vi "Calculate Load Positons from Tube Positions.vi"(7 "PPR":i32=1024, 10 "Tube Counts":i32[](array[numeric])=[47, 213, 383, 557, 724, 898], 11 "Tube Positions":T1[](array[typedef])=[enum."Tube Red A", enum."Tube Black F", enum."Tube Red E", enum."Tube Black D", enum."Tube Red C", enum."Tube Black B"]) -> (2 "Tube Counts Out":i32[](array[numeric]), 3 "Tube Positions Out":T1[](array[typedef]))   [LabVIEW 2023, in "Tube Wheel_ACT.lvlib"]
uses:
  Tube Wheel_ACT.lvlib
  Shared Code/TypeDefs/ENUM_Tube Wheel Positions.ctl
  b52b9a7c-0dc7-454b-b034-c7221ee48ef9.vi
  0a084980-5c52-41c3-8bfb-67c1c4f76a43.vi
  68734bbb-5698-4c3c-834b-1853d34adc1a.vi
  <vilib>/Comparison/Equal/Equal Functor/Equal Functor.lvclass
  <vilib>/Comparison/Less/Less Functor/Less Functor.lvclass
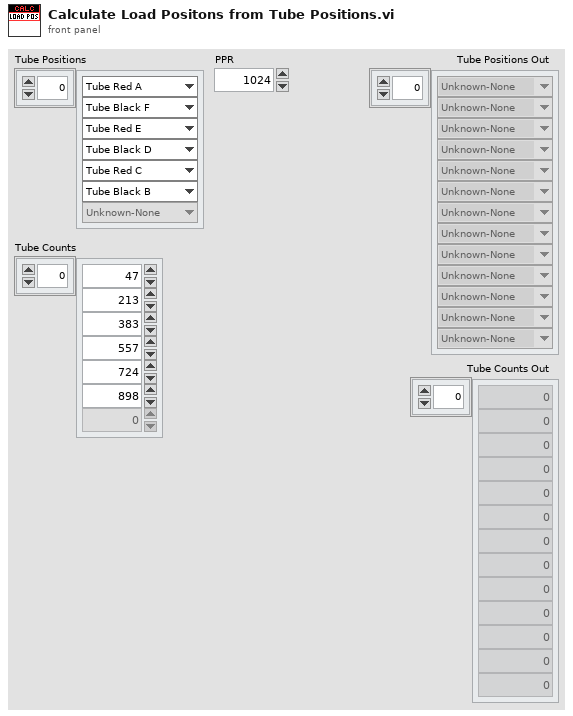
[diagram p1: front panel]
types:
  T1 = typedef "ENUM_Tube Wheel Positions.ctl" = enum16{"Unknown-None", "Tube Red A", "Tube Black B", "Tube Red C", "Tube Black D", "Tube Red E", "Tube Black F", "Load A-B", "Load B-C", "Load C-D", "Load D-E", "Load E-F", "Load F-A"}
  T2 = cluster{"Count":i32, "Tube Wheel Positions":T1}[]
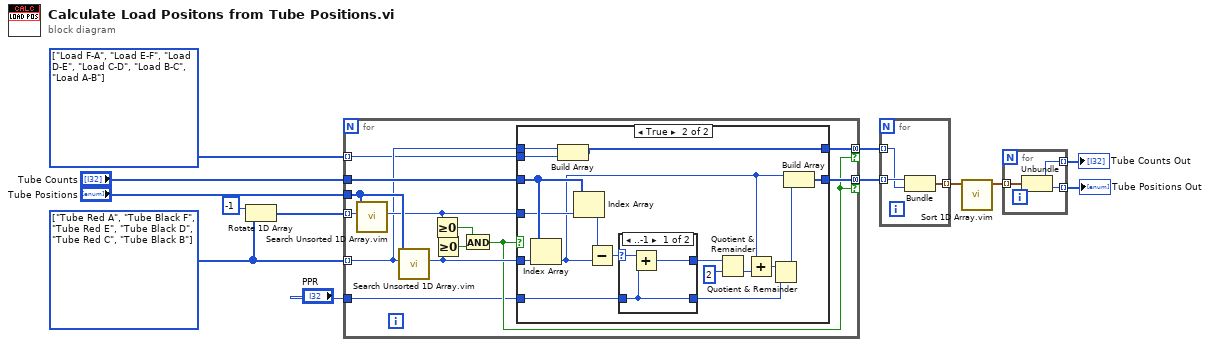
[diagram p0: block diagram]
diagram:
  w10 = T1[] [enum."Load F-A", enum."Load E-F", enum."Load D-E", enum."Load C-D", enum."Load B-C", enum."Load A-B"] items=["Unknown-None", "Tube Red A", "Tube Black B", "Tube Red C", "Tube Black D", "Tube Red E", "Tube Black F", "Load A-B", "Load B-C", "Load C-D", "Load D-E", "Load E-F", "Load F-A"] ("Tube Positions in")
  w12 = T1[] [enum."Tube Red A", enum."Tube Black F", enum."Tube Red E", enum."Tube Black D", enum."Tube Red C", enum."Tube Black B"] items=["Unknown-None", "Tube Red A", "Tube Black B", "Tube Red C", "Tube Black D", "Tube Red E", "Tube Black F", "Load A-B", "Load B-C", "Load C-D", "Load D-E", "Load E-F", "Load F-A"] ("Tube Positions in")
  n1 = Rotate 1D Array(1:w12, 2:-1 ("n")) -> (0:w11:T1[])
  n2 = for {
    tunnel: w12 -> [w19] mode=indexing
    tunnel: w11 -> [w26] mode=indexing
    tunnel: "Tube Positions" -> [w25]
    tunnel: w10 -> [w14] mode=indexing
    tunnel: "Tube Counts" -> [w24]
    tunnel: [w18] -> w7 mode=concatenating if=w16
    tunnel: [w17] -> w6 mode=concatenating if=w16
    tunnel: "PPR" -> [w15]
    n3 = call "Search Unsorted 1D Array.vim"("element"=w26, "unsorted 1D array"=w25) -> ("index of element"=w23:i32)  [unwired: 9 in]
    n4 = call "Search Unsorted 1D Array.vim"("element"=w19, "unsorted 1D array"=w25) -> ("index of element"=w22:i32)  [unwired: 9 in]
    n5 = Greater Or Equal To 0?(x=w23) -> (x >= 0?=w20:bool)
    n6 = Greater Or Equal To 0?(x=w22) -> (x >= 0?=w21:bool)
    n7 = And(x=w20, y=w21) -> (x .and. y?=w16:bool)
    n8 = case shown="True" w16 {
      tunnel: w24 -> [_ w43]
      tunnel: w23 -> [_ w42]
      tunnel: w22 -> [_ w41]
      tunnel: w19 -> [_ w40]
      tunnel: w14 -> [_ w39]
      tunnel: [_ w38] -> w18
      tunnel: [_ w37] -> w17
      tunnel: w15 -> [_ w35]
      frame False {
      }
      frame True {
        n9 = Index Array(array=w43, index=w41) -> (element=w27:i32)
        n10 = Build Array(w40, w39) -> (w38:T1[])
        n11 = Index Array(array=w43, index=w42) -> (element=w28:i32)
        n12 = Subtract(x=w28, y=w27) -> (x-y=w36:i32)
        n13 = case shown="..-1" w36 {
          selector: w36 -> [w46 w48]
          tunnel: [w45 w48] -> w30
          tunnel: w35 -> [w44 w47]
          tunnel: [w44 w47] -> w33
          frame ..-1 {
            n14 = Add(x=w46, y=w44) -> (x+y=w45:i32)
          }
          frame 0.. {
          }
        }
        n15 = Quotient & Remainder(x=w30, y=2) -> (floor(x/y)=w29:i32)  [unwired: 1 out]
        n16 = Add(x=w27, y=w29) -> (x+y=w34:i32)
        n17 = Quotient & Remainder(x=w34, y=w33) -> (x-y*floor(x/y)=w32:i32)  [unwired: 1 out]
        n18 = Build Array(w27, w32) -> (w37:i32[])
      }
    }
  }
  n19 = for {
    tunnel: w7 -> [w50] mode=indexing
    tunnel: w6 -> [w51] mode=indexing
    tunnel: [w49] -> w5 mode=indexing
    n20 = Bundle("Count"=w51, "Tube Wheel Positions"=w50) -> (w49:cluster{"Count":i32, "Tube Wheel Positions":T1})  [unwired: 1 in]
  }
  n21 = call "Sort 1D Array.vim"("unsorted array"=w5) -> ("sorted array"=w4:T2)  [unwired: 10 in]
  n22 = for {
    tunnel: w4 -> [w54] mode=indexing
    tunnel: [w53] -> w1 mode=indexing
    tunnel: [w52] -> w3 mode=indexing
    n23 = Unbundle(w54) -> ("Count"=w53:i32, "Tube Wheel Positions"=w52:T1)
  }
  "Tube Counts Out" <- w1
  "Tube Positions Out" <- w3
